vi "Main.vi"(8 "error in (no error)":errorcluster) -> ()   [LabVIEW 2018]
uses:
  <vilib>/LVH/i3 JSON/JSON Parsing/Get Array Value at Index Files/Get Array Value at Index - Object.vi
  <vilib>/LVH/i3 JSON/JSON Parsing/Get Object Parameter Files/Get Object Parameter - Object.vi
  <vilib>/LVH/i3 JSON/JSON Parsing/Get Object Parameter Files/Get Object Parameter - String.vi
  <vilib>/LVH/i3 JSON/JSON Parsing/Get Array Value at Index Files/Get Array Value at Index - String.vi
  <vilib>/httpClient/LabVIEWHTTPClient.lvlib
  <vilib>/LVH/i3 JSON/i3-json.lvlib
panel:
  out "body":string
  out "Sound Found?":bool
  out "Output":string
  in  "Simulate?":bool
  out "Random Word":string
  out "Origin":string
  in  "Play Sound?":bool
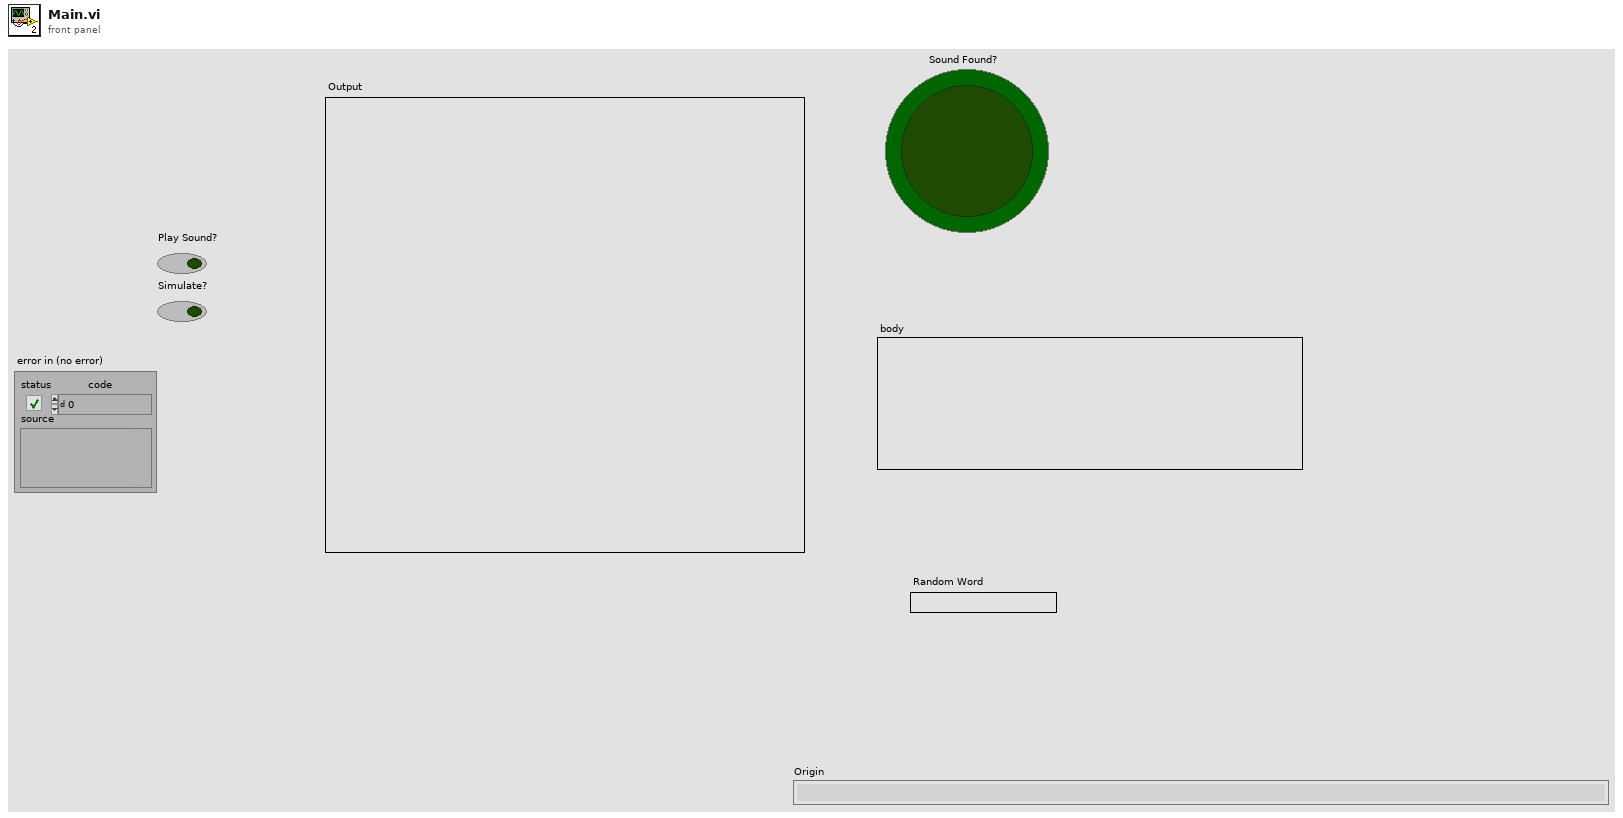
[diagram p1: front panel]
types:
  T1 = cluster{"mw":string, "l":string, "l2":string, "pun":string, "sound":cluster{"audio":string, "ref":string, "stat":string}}
  T2 = cluster{"id":string, "uuid":string, "sort":string, "src":string, "section":string, "stems":string[], "offensive":bool}
  T3 = typedef "LabVIEWHTTPClient.lvlib/ClientHandle.ctl" = refnum<k1>
  T4 = enum16{"open", "replace", "create", "open or create", "replace or create", "replace or create with confirmation"}
  T5 = typedef "Sound Output Task ID.ctl" = u32
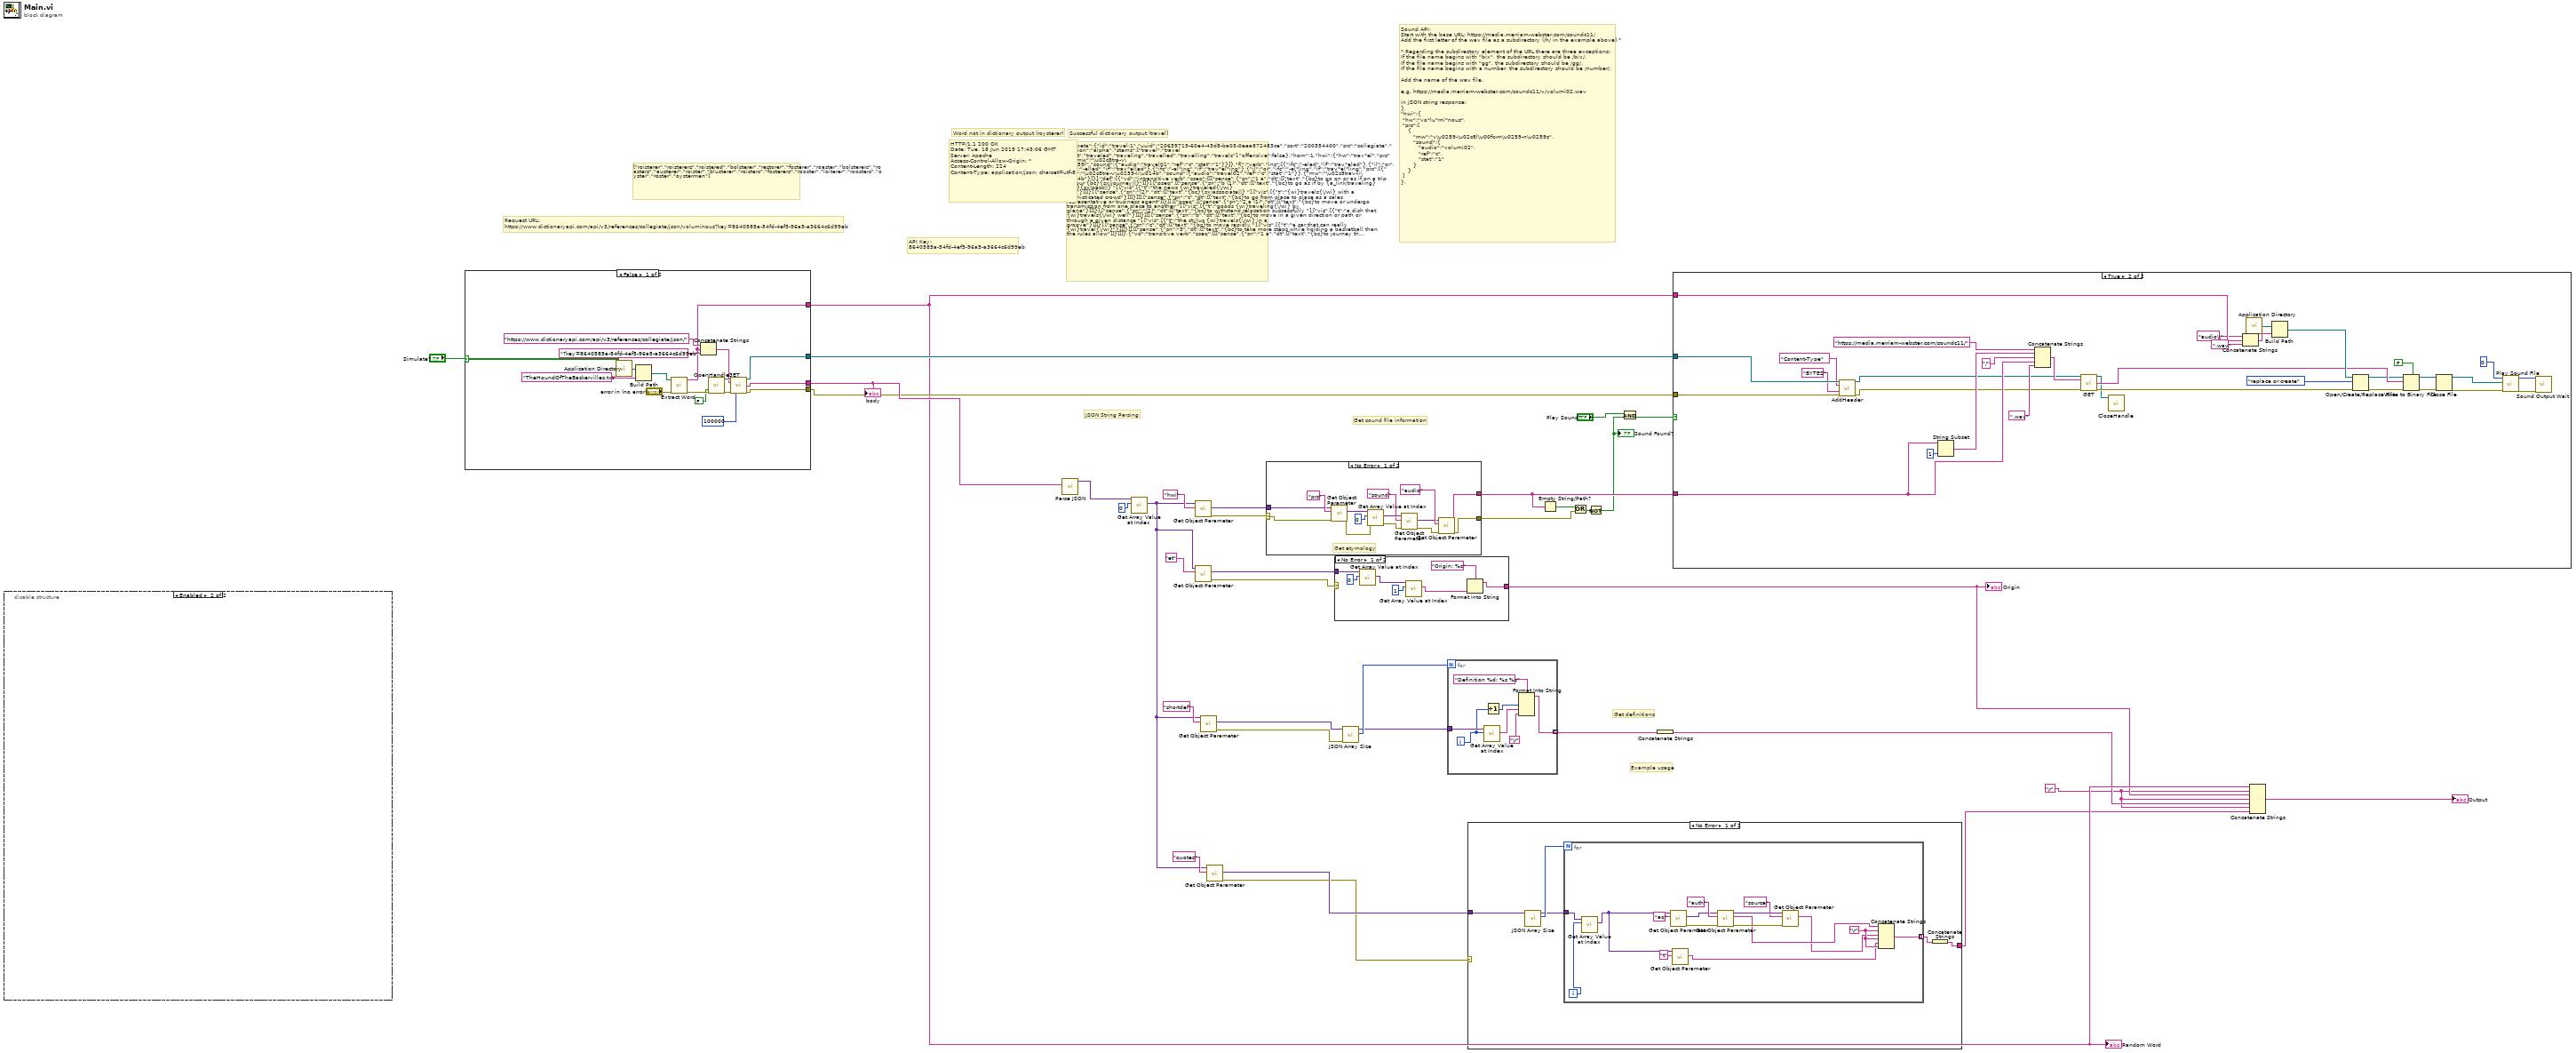
[diagram p0: block diagram]
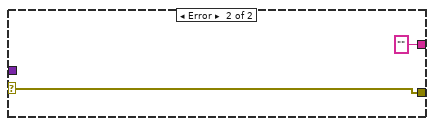
[diagram p2: hidden frame]
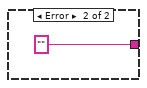
[diagram p3: hidden frame]
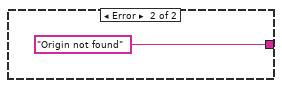
[diagram p4: hidden frame]
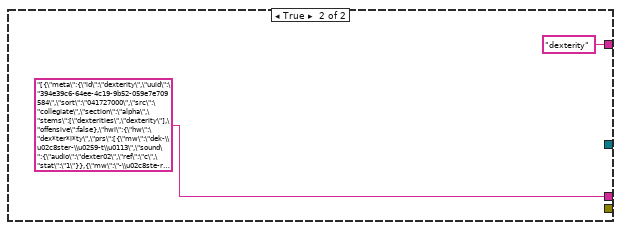
[diagram p5: hidden frame]
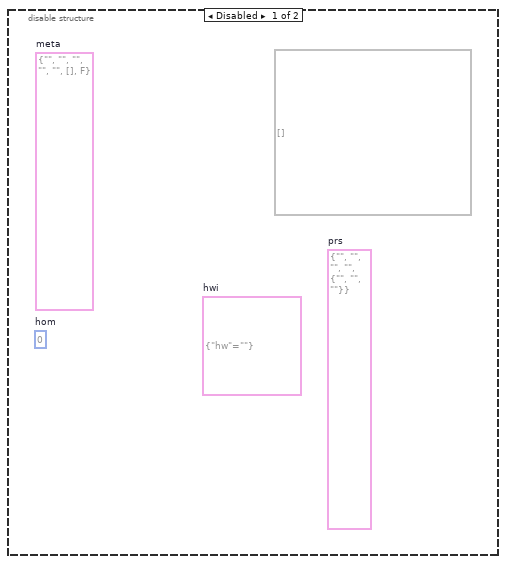
[diagram p6: hidden frame]
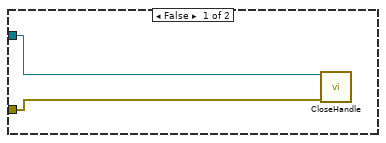
[diagram p7: hidden frame]
diagram:
  w9 = "\r"
  # "Example usage"
  # "Get definitions"
  # "Get sound file information"
  # "JSON String Parsing"
  # "Successful dictionary output (travel)"
  # "[{\"meta\":{\"id\":\"travel:1\",\"uuid\":\"20639719-60e4-43d8-ba03-0eea872483ce\",\"sort\":\"200354400\",\"src\":\"collegiate\",\"section\":\"alpha\",\"stems\":[\"travel\",\"travel light\",\"traveled\",\"traveling\",\"travelled\",\"travelling\",\"travels\"],\"offensive\":false},\"hom\":1,\"hwi\":{\"hw\":\"trav*el\",\"prs\":[{\"mw\":\"\\u02c8tra-v\\u0259l\",\"sound\":{\"audio\":\"travel01\",\"ref\":\"c\",\"stat\":\"1\"}}]},\"fl\":\"verb\",\"ins\":[{\"ifc\":\"-eled\",\"if\":\"trav*eled\"},{\"il\":\"or\",\"ifc\":\"-elled\",\"if\":\"trav*elled\"},{\"ifc\":\"-el*ing\",\"if\":\"trav*el*ing\"},{\"il\":\"or\",\"ifc\":\"-el*ling\",\"if\":\"trav*el*ling\",\"prs\":[{\"mw\":\"\\u02c8tra-v\\u0259-li\\u014b\",\"sound\":{\"audio\":\"travel02\",\"ref\":\"c\",\"stat\":\"1\"}},{\"mw\":\"\\u02c8trav-li\\u014b\"}]}],\"def\":[{\"vd\":\"intransitive verb\",\"sseq\":[[[\"sense\",{\"sn\":\"1 a\",\"dt\":[[\"text\",\"{bc}to go on or as if on a trip or tour {bc}{sx|journey||}\"]]}],[\"pseq\",[[\"sense\",{\"sn\":\"b (1)\",\"dt\":[[\"text\",\"{bc}to go as if by {a_link|traveling} {bc}{sx|pass||} \"],[\"vis\",[{\"t\":\"the news {wi}traveled{\\/wi} fast\"}]]]}],[\"sense\",{\"sn\":\"(2)\",\"dt\":[[\"text\",\"{bc}{sx|associate||} \"],[\"vis\",[{\"t\":\"{wi}travels{\\/wi} with a sophisticated crowd\"}]]]}]]],[\"sense\",{\"sn\":\"c\",\"dt\":[[\"text\",\"{bc}to go from place to place as a sales representative or business agent\"]]}]],[[\"pseq\",[[\"sense\",{\"sn\":\"2 a (1)\",\"dt\":[[\"text\",\"{bc}to move or undergo transmission from one place to another \"],[\"vis\",[{\"t\":\"goods {wi}traveling{\\/wi} by plane\"}]]]}],[\"sense\",{\"sn\":\"(2)\",\"dt\":[[\"text\",\"{bc}to withstand relocation successfully \"],[\"vis\",[{\"t\":\"a dish that {wi}travels{\\/wi} well\"}]]]}]]],[\"sense\",{\"sn\":\"b\",\"dt\":[[\"text\",\"{bc}to move in a given direction or path or through a given distance \"],[\"vis\",[{\"t\":\"the stylus {wi}travels{\\/wi} in a groove\"}]]]}],[\"sense\",{\"sn\":\"c\",\"dt\":[[\"text\",\"{bc}to move rapidly \"],[\"vis\",[{\"t\":\"a car that can really {wi}travel{\\/wi}\"}]]]}]],[[\"sense\",{\"sn\":\"3\",\"dt\":[[\"text\",\"{bc}to take more steps while holding a basketball than the rules allow\"]]}]]]},{\"vd\":\"transitive verb\",\"sseq\":[[[\"sense\",{\"sn\":\"1 a\",\"dt\":[[\"text\",\"{bc}to journey through or over\"]]}],[\"sense\",{\"sn\":\"b\",\"dt\":[[\"text\",\"{bc}to follow (a course or path) as if by traveling\"]]}]],[[\"sense\",{\"sn\":\"2\",\"dt\":[[\"text\",\"{bc}to {a_link|traverse} (a specified distance)\"]]}]],[[\"sense\",{\"sn\":\"3\",\"dt\":[[\"text\",\"{bc}to cover (an area) as a commercial {a_link|traveler}\"]]}]]]}],\"dros\":[{\"drp\":\"travel light\",\"def\":[{\"sseq\":[[[\"sense\",{\"dt\":[[\"text\",\"{bc}to travel with a minimum of equipment or baggage\"]]}]]]}]}],\"et\":[[\"text\",\"Middle English {it}travailen, travelen{\\/it} to torment, labor, strive, journey, from Anglo-French {it}travailler{\\/it}\"]],\"date\":\"14th century{ds|i|1|a|}\",\"shortdef\":[\"to go on or as if on a trip or tour : journey\",\"to go as if by traveling : pass\",\"associate\"]},{\"meta\":{\"id\":\"travel:2\",\"uuid\":\"ab8700b4-a3f0-43b6-b9bb-c96188bab682\",\"sort\":\"200354500\",\"src\":\"collegiate\",\"section\":\"alpha\",\"stems\":[\"travel\",\"travels\"],\"offensive\":false},\"hom\":2,\"hwi\":{\"hw\":\"travel\"},\"fl\":\"noun\",\"def\":[{\"sseq\":[[[\"sense\",{\"sn\":\"1 a\",\"dt\":[[\"text\",\"{bc}the act of {a_link|traveling} {bc}{sx|passage||}\"]]}],[\"sense\",{\"sn\":\"b\",\"dt\":[[\"text\",\"{bc}a journey especially to a distant or unfamiliar place {bc}{sx|tour||}, {sx|trip||} \"],[\"uns\",[[[\"text\",\"often used in plural\"]]]]]}]],[[\"sense\",{\"sn\":\"2\",\"ins\":[{\"if\":\"trav*els\",\"spl\":\"plural\"}],\"dt\":[[\"text\",\"{bc}an account of one\\u0027s {a_link|travels}\"]]}]],[[\"sense\",{\"sn\":\"3\",\"dt\":[[\"text\",\"{bc}the number traveling {bc}{sx|traffic||}\"]]}]],[[\"sense\",{\"sn\":\"4 a\",\"dt\":[[\"text\",\"{bc}{sx|movement||}, {sx|progression||} \"],[\"vis\",[{\"t\":\"the {wi}travel{\\/wi} of satellites around the earth\"}]]]}],[\"sense\",{\"sn\":\"b\",\"dt\":[[\"text\",\"{bc}the motion of a piece of machinery\"]],\"sdsense\":{\"sd\":\"especially\",\"dt\":[[\"text\",\"{bc}reciprocating motion\"]]}}]]]}],\"date\":\"14th century{ds||1|a|}\",\"shortdef\":[\"the act of traveling : passage\",\"a journey especially to a distant or unfamiliar place : tour, trip \\u2014often used in plural\",\"an account of one\\u0027s travels\"]},{\"meta\":{\"id\":\"travel agency\",\"uuid\":\"6acf6088-0890-46e7-8515-41ac48fa5358\",\"sort\":\"200354600\",\"src\":\"collegiate\",\"section\":\"alpha\",\"stems\":[\"travel agencies\",\"travel agency\",\"travel bureau\"],\"offensive\":false},\"hwi\":{\"hw\":\"travel agency\"},\"fl\":\"noun\",\"def\":[{\"sseq\":[[[\"sense\",{\"dt\":[[\"text\",\"{bc}an agency engaged in selling and arranging transportation, accommodations, tours, and trips for travelers \"],[\"ca\",{\"intro\":\"called also\",\"cats\":[{\"cat\":\"travel bureau\"}]}]]}]]]}],\"date\":\"1927\",\"shortdef\":[\"an agency engaged in selling and arranging transportation, accommodations, tours, and trips for travelers \\u2014called also travel bureau\"]},{\"meta\":{\"id\":\"travel agent\",\"uuid\":\"da18f052-f396-446b-a328-e046d94b928c\",\"sort\":\"200354700\",\"src\":\"collegiate\",\"section\":\"alpha\",\"stems\":[\"travel agent\",\"travel agents\"],\"offensive\":false},\"hwi\":{\"hw\":\"travel agent\"},\"fl\":\"noun\",\"def\":[{\"sseq\":[[[\"sense\",{\"dt\":[[\"text\",\"{bc}a person engaged in selling and arranging transportation, accommodations, tours, or trips for travelers\"]]}]]]}],\"date\":\"1925\",\"shortdef\":[\"a person engaged in selling and arranging transportation, accommodations, tours, or trips for travelers\"]},{\"meta\":{\"id\":\"travel bag\",\"uuid\":\"07856c26-afc9-4e1a-a5f9-e3b1b19cc97a\",\"sort\":\"200354750\",\"src\":\"collegiate\",\"section\":\"alpha\",\"stems\":[\"travel bag\",\"travel bags\",\"traveling bag\",\"traveling bags\"],\"offensive\":false},\"hwi\":{\"hw\":\"travel bag\"},\"vrs\":[{\"vl\":\"or\",\"va\":\"traveling bag\"}],\"fl\":\"noun\",\"def\":[{\"sseq\":[[[\"sense\",{\"dt\":[[\"text\",\"{bc}{sx|suitcase||}\"]]}]]]}],\"date\":\"1826\",\"shortdef\":[\"suitcase\"]},{\"meta\":{\"id\":\"travel trailer\",\"uuid\":\"7105ccd6-15cf-4979-8b02-51a1b2fc6731\",\"sort\":\"200355800\",\"src\":\"collegiate\",\"section\":\"alpha\",\"stems\":[\"travel trailer\",\"travel trailers\"],\"offensive\":false},\"hwi\":{\"hw\":\"travel trailer\"},\"fl\":\"noun\",\"def\":[{\"sseq\":[[[\"sense\",{\"dt\":[[\"text\",\"{bc}a trailer drawn especially by an automobile and equipped for use (as while traveling) as a dwelling\"]]}]]]}],\"date\":\"1961\",\"shortdef\":[\"a trailer drawn especially by an automobile and equipped for use (as while traveling) as a dwelling\"]},{\"meta\":{\"id\":\"travel sickness\",\"uuid\":\"105d0afa-84f0-492e-bb85-58715df92456\",\"sort\":\"3021430000\",\"src\":\"ld\",\"section\":\"idioms\",\"stems\":[\"travel sickness\"],\"offensive\":false},\"hwi\":{\"hw\":\"travel sickness\"},\"fl\":\"noun\",\"def\":[{\"sls\":[\"British\"],\"sseq\":[[[\"sense\",{\"dt\":[[\"text\",\"{bc}a feeling of sickness caused by the motion of a car, airplane, boat, etc.\"]]}]]]}],\"shortdef\":[\"a feeling of sickness caused by the motion of a car, airplane, boat, etc.\"]},{\"meta\":{\"id\":\"pretravel\",\"uuid\":\"9980ad5e-be76-42a8-b754-9dc0105550aa\",\"sort\":\"162336000\",\"src\":\"collegiate\",\"section\":\"alpha\",\"stems\":[\"pre-travel\",\"pretravel\"],\"offensive\":false},\"hwi\":{\"hw\":\"pre*trav*el\",\"prs\":[{\"mw\":\"\\u02ccpr\\u0113-\\u02c8tra-v\\u0259l\",\"sound\":{\"audio\":\"pretravel_1\",\"ref\":\"owl\",\"stat\":\"1\"}}]},\"vrs\":[{\"vl\":\"or\",\"va\":\"pre-travel\"}],\"fl\":\"adjective\",\"def\":[{\"sseq\":[[[\"sense\",{\"dt\":[[\"text\",\"{bc}before {d_link|travel|travel:1} {bc}occurring or existing prior to travelling \"],[\"vis\",[{\"t\":\"{wi}pretravel{\\/wi} planning\"},{\"t\":\"a {wi}pretravel{\\/wi} medical consultation\"}]]]}]]]}],\"date\":\"1915\",\"shortdef\":[\"before travel : occurring or existing prior to travelling\"]},{\"meta\":{\"id\":\"the world\",\"uuid\":\"6c5a6e9a-715d-4ea8-a311-271f67d2de3d\",\"sort\":\"3020748000\",\"src\":\"ld\",\"section\":\"idioms\",\"stems\":[\"the world\",\"halfway around\\/across the world\",\"halfway across the world\",\"halfway around the world\",\"the rest of the world\",\"see\\/travel the world\",\"see the world\",\"travel the world\",\"the eyes of the world\"],\"offensive\":false},\"hwi\":{\"hw\":\"the world\"},\"fl\":\"noun\",\"def\":[{\"sseq\":[[[\"sense\",{\"sn\":\"1\",\"dt\":[[\"text\",\"{bc}the earth and all the people and things on it \"],[\"vis\",[{\"t\":\"He is famous throughout {it}the world{\\/it}.\"},{\"t\":\"They sailed around {it}the world{\\/it}.\"},{\"t\":\"The product is shipped {phrase}halfway around\\/across the world{\\/phrase}.\"},{\"t\":\"The island was cut off from {phrase}the rest of the world{\\/phrase}.\"},{\"t\":\"They want to {phrase}see\\/travel the world{\\/phrase}.\"}]]]}]],[[\"sense\",{\"sn\":\"2\",\"dt\":[[\"text\",\"{bc}the people in the world \"],[\"vis\",[{\"t\":\"She felt that {it}the world{\\/it} was against her.\"},{\"t\":\"They announced their discovery to {it}the world{\\/it}.\"},{\"t\":\"{it}The world{\\/it} watched as he attempted to break the Olympic record.\"},{\"t\":\"She felt {phrase}the eyes of the world{\\/phrase} watching her.\"}]]]}]],[[\"sense\",{\"sn\":\"3\",\"dt\":[[\"text\",\"{bc}all that is important {bc}everything \"],[\"vis\",[{\"t\":\"I would give my children {it}the world{\\/it} if I could.\"}]]]}]]]}],\"shortdef\":[\"the earth and all the people and things on it\",\"the people in the world\",\"all that is important : everything\"]}]"
  # "[\"roisterer\",\"roisterers\",\"roistered\",\"bolsterer\",\"restorer\",\"fosterer\",\"roaster\",\"bolsterers\",\"roasters\",\"austerer\",\"roister\",\"blusterer\",\"roisters\",\"fosterers\",\"rooster\",\"loiterer\",\"roosters\",\"oyster\",\"roster\",\"oystermen\"]"
  # "Word not in dictionary output (roysterer)"
  # "HTTP/1.1 200 OK\nDate: Tue, 18 Jun 2019 17:43:06 GMT\nServer: Apache\nAccess-Control-Allow-Origin: *\nContent-Length: 224\nContent-Type: application/json; charset=utf-8"
  # "API Key:\n8640585a-54fd-4ef5-96a5-a3664c6d99eb"
  # "Request URL:\nhttps://www.dictionaryapi.com/api/v3/references/collegiate/json/voluminous?key=8640585a-54fd-4ef5-96a5-a3664c6d99eb"
  # "Sound API:\nStart with the base URL: https://media.merriam-webster.com/soundc11/\nAdd the first letter of the wav file as a subdirectory (/h/ in the example above).*\n\n* Regarding the subdirectory element of the URL there are three exceptions:\nIf the file name begins with \"bix\", the subdirectory should be /bix/.\nIf the file name begins with \"gg\", the subdirectory should be /gg/.\nIf the file name begins with a number, the subdirectory should be /number/.\n\nAdd the name of the wav file.\n\ne.g. https://media.merriam-webster.com/soundc11/v/volumi02.wav\n\nin JSON string response:\n},\n\"hwi\":{  \n \"hw\":\"vo*lu*mi*nous\",\n \"prs\":[  \n    {  \n       \"mw\":\"v\\u0259-\\u02c8l\\u00fc-m\\u0259-n\\u0259s\",\n       \"sound\":{  \n          \"audio\":\"volumi02\",\n          \"ref\":\"c\",\n          \"stat\":\"1\"\n       }\n    }\n ]\n},"
  n1 = disable-structure shown="Enabled" {
    frame Disabled {
      (unwired) T1 {"mw"="", "l"="", "l2"="", "pun"="", "sound"={"audio"="", "ref"="", "stat"=""}}  # prs
      (unwired) void[] []
      (unwired) cluster{"hw":string} {"hw"=""}  # hwi
      (unwired) 0  # hom
      (unwired) T2 {"id"="", "uuid"="", "sort"="", "src"="", "section"="", "stems"=[], "offensive"=FALSE}  # meta
    }
    frame Enabled {
    }
  }
  n2 = case shown="False" "Simulate?" {
    tunnel: [w40 _] -> w25
    tunnel: [w39 _] -> w24
    tunnel: [w36 "dexterity" ("Random Word")] -> w13
    tunnel: [w37 "[{\"meta\":{\"id\":\"dexterity\",\"uuid\":\"394e39c6-64ee-4c19-9b52-059e7e709584\",\"sort\":\"041727000\",\"src\":\"collegiate\",\"section\":\"alpha\",\"stems\":[\"dexterities\",\"dexterity\"],\"offensive\":false},\"hwi\":{\"hw\":\"dex*ter*i*ty\",\"prs\":[{\"mw\":\"dek-\\u02c8ster-\\u0259-t\\u0113\",\"sound\":{\"audio\":\"dexter02\",\"ref\":\"c\",\"stat\":\"1\"}},{\"mw\":\"-\\u02c8ste-r\\u0259-\"}]},\"fl\":\"noun\",\"ins\":[{\"il\":\"plural\",\"ifc\":\"-ties\",\"if\":\"dex*ter*i*ties\"}],\"def\":[{\"sseq\":[[[\"sense\",{\"sn\":\"1\",\"dt\":[[\"text\",\"{bc}readiness and {d_link|grace|grace:1} in physical activity\"]],\"sdsense\":{\"sd\":\"especially\",\"dt\":[[\"text\",\"{bc}skill and ease in using the hands \"],[\"vis\",[{\"t\":\"manual {wi}dexterity{\\/wi}\"}]]]}}]],[[\"sense\",{\"sn\":\"2\",\"dt\":[[\"text\",\"{bc}mental skill or quickness {bc}{sx|adroitness||}\"]]}]]]}],\"quotes\":[{\"t\":\"Russ Cellan, Ferguson\\u0027s coach at Freeport (New York) High, and Ron Prince, his former offensive line coach at Virginia, both attribute Ferguson\\u0027s {qword}dexterity{\\/qword} and footwork to his extensive martial arts training \\u2026\",\"aq\":{\"auth\":\"Nunyo Demasio\",\"source\":\"{it}Sports Illustrated{\\/it}\",\"aqdate\":\"10 Apr. 2006\"}},{\"t\":\"The Carcanet volume also offers its readers the advantage of seeing the German originals alongside the English, enabling them to perceive at a glance how much sympathy and linguistic {qword}dexterity{\\/qword} Elliot has brought to the difficult but rewarding task of introducing a new generation of English readers to Heine\\u0027s tragic but wonderfully vigorous and vivid late poetry.\",\"aq\":{\"auth\":\"S. S. Prawer\",\"source\":\"{it}Times Literary Supplement{\\/it}\",\"aqdate\":\"28 Sept. - 4 Oct. 1990\"}},{\"t\":\"But the mayor showed considerable political {qword}dexterity{\\/qword} in the days following the fire, taking care to distance himself from on-site decisions while accepting full responsibility for the bombing itself. He made himself available to reporters, met with people from the fire-ravaged neighborhood, and was gracious enough not to blame subordinates.\",\"aq\":{\"auth\":\"Amy Wilentz\",\"source\":\"{it}Time{\\/it}\",\"aqdate\":\"27 May 1985\"}}],\"et\":[[\"text\",\"Middle French or Latin; Middle French {it}dexterit\\u00e9{\\/it}, from Latin {it}dexteritat-, dexteritas{\\/it}, from {it}dexter{\\/it} {dx_ety}see {dxt|dexterous||}{\\/dx_ety}\"]],\"date\":\"1518{ds||2||}\",\"shortdef\":[\"readiness and grace in physical activity; especially : skill and ease in using the hands\",\"mental skill or quickness : adroitness\"]}]"] -> w30
    frame False {
      n3 = call <vilib>:"Application Directory.vi"() -> ("Application Directory"=w50:path)
      n4 = Build Path(base path=w50, name or relative path="TheHoundOfTheBaskervilles.txt") -> (appended path=w48:path)
      n5 = call "Extract Word.vi"("error in (no error)"="error in (no error)", "file path (use dialog)"=w48) -> ("error out"=w47:errorcluster, "Random Word"=w36:string)  [unwired: 8 in]
      n6 = Concatenate Strings("https://www.dictionaryapi.com/api/v3/references/collegiate/json/" ("string"), w36, "?key=8640585a-54fd-4ef5-96a5-a3664c6d99eb") -> (w42:string)
      n7 = call <vilib>:"OpenHandle.vi"("error in (no error)"=w47, "verify server(true)"=FALSE) -> ("client handle out"=w46:T3, "error out"=w45:errorcluster)  [unwired: 12 in]
      n8 = call <vilib>:"GET.vi"("client handle"=w46, "url"=w42, "error in (no error)"=w45, "timeout (10000)"=100000) -> ("client handle out"=w40:T3, "body"=w37:string, "error out"=w39:errorcluster)  [unwired: 8 in, 1 out]
    }
    frame True {
    }
  }
  "Random Word" <- w13
  "body" <- w30
  n9 = call <vilib>:"Parse JSON.vi"("JSON String"=w30) -> ("JSON Tree"=w35:variant)  [unwired: 7 in, 3 out]
  n10 = call-poly <vilib>:"Get Array Value at Index.vi"("Index"=0, "JSON Tree In (JSON Array)"=w35) -> ("JSON Object"=w17:variant)  [unwired: 6 in, 3 out]
  n11 = call-poly <vilib>:"Get Object Parameter.vi"("Parameter Name"="hwi", "JSON Tree In (JSON Object)"=w17) -> ("error out"=w7:errorcluster, "JSON Object"=w32:variant)  [unwired: 6 in, 2 out]
  n12 = call-poly <vilib>:"Get Object Parameter.vi"("Parameter Name"="et", "JSON Tree In (JSON Object)"=w17) -> ("error out"=w23:errorcluster, "JSON Object"=w28:variant)  [unwired: 6 in, 2 out]
  n13 = call-poly <vilib>:"Get Object Parameter.vi"("Parameter Name"="shortdef", "JSON Tree In (JSON Object)"=w17) -> ("error out"=w19:errorcluster, "JSON Object"=w22:variant)  [unwired: 6 in, 2 out]
  n14 = call-poly <vilib>:"Get Object Parameter.vi"("Parameter Name"="quotes", "JSON Tree In (JSON Object)"=w17) -> ("error out"=w15:errorcluster, "JSON Object"=w16:variant)  [unwired: 6 in, 2 out]
  n15 = case shown="No Error" w7 {
    selector: w7 -> [w58 w68]
    tunnel: w32 -> [w61 _]
    tunnel: [w59 "" ("String Value")] -> w6
    tunnel: [w54 w68] -> w4
    frame No Error {
      # "Get etymology"
      n16 = call-poly <vilib>:"Get Object Parameter.vi"("error in (no error)"=w58, "Parameter Name"="prs", "JSON Tree In (JSON Object)"=w61) -> ("error out"=w57:errorcluster, "JSON Object"=w60:variant)  [unwired: 5 in, 2 out]
      n17 = call-poly <vilib>:"Get Array Value at Index.vi"("error in (no error)"=w57, "Index"=0, "JSON Tree In (JSON Array)"=w60) -> ("error out"=w56:errorcluster, "JSON Object"=w66:variant)  [unwired: 5 in, 2 out]
      n18 = call-poly <vilib>:"Get Object Parameter.vi"("error in (no error)"=w56, "Parameter Name"="sound", "JSON Tree In (JSON Object)"=w66) -> ("error out"=w55:errorcluster, "JSON Object"=w63:variant)  [unwired: 5 in, 2 out]
      n19 = call-poly <vilib>:"Get Object Parameter.vi"("error in (no error)"=w55, "Parameter Name"="audio", "JSON Tree In (JSON Object)"=w63) -> ("error out"=w54:errorcluster, "String Value"=w59:string)  [unwired: 5 in, 2 out]
    }
    frame Error {
    }
  }
  n20 = case shown="No Error" w23 {
    tunnel: w28 -> [w75 _]
    tunnel: [w70 "Origin not found" ("String Value")] -> w12
    frame No Error {
      n21 = call-poly <vilib>:"Get Array Value at Index.vi"("Index"=0, "JSON Tree In (JSON Array)"=w75) -> ("JSON Object"=w73:variant)  [unwired: 6 in, 3 out]
      n22 = call-poly <vilib>:"Get Array Value at Index.vi"("Index"=1, "JSON Tree In (JSON Array)"=w73) -> ("String Value"=w72:string)  [unwired: 6 in, 3 out]
      n23 = Format Into String(format string="Origin: %s", w72) -> (resulting string=w70:string)  [unwired: 2 in, 1 out]
    }
    frame Error {
    }
  }
  "Origin" <- w12
  n24 = call <vilib>:"JSON Array Size.vi"("error in (no error)"=w19, "JSON Tree In (JSON Array)"=w22) -> ("Array Size"=w21:i32, "JSON Tree Passthrough (JSON Array)"=w20:variant)  [unwired: 7 in, 1 out]
  n25 = for {
    N: w21 -> [_]
    tunnel: w20 -> [w84]
    tunnel: [w78] -> w14 mode=indexing
    i -> [w82]
    n26 = call-poly <vilib>:"Get Array Value at Index.vi"("Index"=w82, "JSON Tree In (JSON Array)"=w84) -> ("String Value"=w80:string)  [unwired: 6 in, 3 out]
    n27 = Increment(x=w82) -> (x+1=w81:i32)
    n28 = Format Into String(format string="Definition %d: %s %s", w81, w80, "\r") -> (resulting string=w78:string)  [unwired: 2 in, 1 out]
  }
  n29 = case shown="No Error" w15 {
    tunnel: w16 -> [w89 _]
    tunnel: [w85 ""] -> w10
    frame No Error {
      n30 = call <vilib>:"JSON Array Size.vi"("JSON Tree In (JSON Array)"=w89) -> ("Array Size"=w88:i32, "JSON Tree Passthrough (JSON Array)"=w87:variant)  [unwired: 8 in, 1 out]
      n31 = for {
        N: w88 -> [_]
        tunnel: w87 -> [w97]
        tunnel: [w90] -> w86 mode=indexing
        i -> [w96]
        w94 = "\r"
        n32 = call-poly <vilib>:"Get Array Value at Index.vi"("Index"=w96, "JSON Tree In (JSON Array)"=w97) -> ("JSON Object"=w95:variant)  [unwired: 6 in, 3 out]
        n33 = call-poly <vilib>:"Get Object Parameter.vi"("Parameter Name"="aq", "JSON Tree In (JSON Object)"=w95) -> ("error out"=w99:errorcluster, "JSON Object"=w100:variant)  [unwired: 6 in, 2 out]
        n34 = call-poly <vilib>:"Get Object Parameter.vi"("Parameter Name"="t", "JSON Tree In (JSON Object)"=w95) -> ("String Value"=w91:string)  [unwired: 6 in, 3 out]
        n35 = call-poly <vilib>:"Get Object Parameter.vi"("error in (no error)"=w99, "Parameter Name"="auth", "JSON Tree In (JSON Object)"=w100) -> ("error out"=w102:errorcluster, "String Value"=w93:string, "JSON Tree Out Passthrough"=w104:variant)  [unwired: 5 in, 1 out]
        n36 = call-poly <vilib>:"Get Object Parameter.vi"("error in (no error)"=w102, "Parameter Name"="source", "JSON Tree In (JSON Object)"=w104) -> ("String Value"=w92:string)  [unwired: 5 in, 3 out]
        n37 = Concatenate Strings(w93, w94, w92, w94, w91, w94) -> (w90:string)
      }
      n38 = Concatenate Strings(w86) -> (w85:string)
    }
    frame Error {
    }
  }
  n39 = Empty String/Path?(string/path=w6) -> (empty?=w3:bool)
  n40 = Or(x=w3, y=w4) -> (x .or. y?=w5:bool)
  n41 = Not(x=w5) -> (.not. x?=w1:bool)
  "Sound Found?" <- w1
  n42 = And(x="Play Sound?", y=w1) -> (x .and. y?=w2:bool)
  n43 = Concatenate Strings(w14) -> (w11:string)
  n44 = case shown="True" w2 {
    tunnel: w13 -> [_ w141]
    tunnel: w6 -> [_ w132]
    tunnel: w25 -> [w108 w114]
    tunnel: w24 -> [w107 w111]
    frame False {
      n45 = call <vilib>:"CloseHandle.vi"("client handle"=w108, "error in (no error)"=w107) -> ()  [unwired: 13 in, 1 out]
    }
    frame True {
      n46 = call <vilib>:"AddHeader.vi"("client handle"=w114, "header"="Content-Type", "value"="BYTES", "error in (no error)"=w111) -> ("client handle out"=w110:T3, "error out"=w109:errorcluster)  [unwired: 10 in]
      n47 = String Subset(string=w132, length (rest)=1 ("length (rest)")) -> (substring=w134:string)  [unwired: 1 in]
      n48 = Concatenate Strings("https://media.merriam-webster.com/soundc11/" ("url"), w134, "/" ("string"), w132, ".wav") -> (w130:string)
      n49 = call <vilib>:"GET.vi"("client handle"=w110, "url"=w130, "error in (no error)"=w109) -> ("client handle out"=w115:T3, "body"=w137:string, "error out"=w138:errorcluster)  [unwired: 9 in, 1 out]
      n50 = call <vilib>:"CloseHandle.vi"("client handle"=w115) -> ()  [unwired: 14 in, 1 out]
      n51 = Concatenate Strings("audio\\" ("name or relative path"), w141, ".wav" ("string")) -> (w117:string)
      n52 = call <vilib>:"Application Directory.vi"() -> ("Application Directory"=w119:path)
      n53 = Build Path(base path=w119, name or relative path=w117) -> (appended path=w140:path)
      n54 = Open/Create/Replace File(file path (use dialog)=w140, error in=w138, operation (0:open)=T4."replace or create") -> (refnum out=w129:refnum<file>, error out=w128:errorcluster)  [unwired: 3 in, 1 out]
      n55 = Write to Binary File(file (use dialog)=w129, data=w137, error in=w128, 5:FALSE ("prepend array or string size? (T)")) -> (refnum out=w127:refnum<file>, error out=w126:errorcluster)  [unwired: 2 in, 1 out]
      n56 = Close File(refnum=w127, error in=w126) -> (path=w124:path, error out=w123:errorcluster)
      n57 = call <vilib>:"Play Sound File.vi"("error in (no error)"=w123, "path"=w124, "device ID"=u32 0) -> ("error out"=w120:errorcluster, "task ID"=w121:T5)  [unwired: 7 in]
      n58 = call <vilib>:"Sound Output Wait.vi"("error in (no error)"=w120, "task ID"=w121) -> ()  [unwired: 8 in, 2 out]
    }
  }
  n59 = Concatenate Strings(w13, w9, w12, w9, w11, w9, w10) -> (→"Output":string)
